vi "Plugin.Initialize.vi"(8 "error in (no error)":errorcluster, 10 "Transfers":refnum<class "DSF.Engine.Transfer.lvclass">[](array[class]), 11 "UDP Plugin in":refnum<class "UDP Plugin.lvclass">) -> (0 "error out":errorcluster, 3 "UDP Plugin out":refnum<class "UDP Plugin.lvclass">)   [LabVIEW 2017, in "UDP Plugin.lvclass"]
uses:
  UDP Plugin.lvclass
  Source/Engine/Classes/Transfer/DSF.Engine.Transfer.lvclass
  UDP Plugin.lvclass/UDP Plugin.ctl
  Source/Engine/Classes/Transfer/DSF.Engine.Transfer.lvclass/DSF.Engine.Transfer.ctl
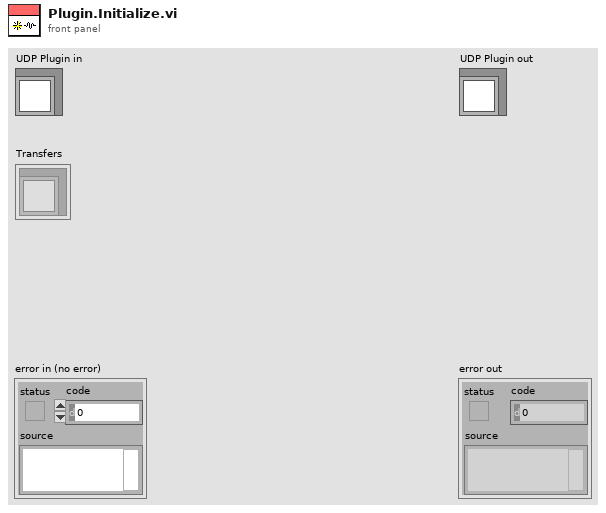
[diagram p1: front panel]
types:
  T1 = typedef "DSF.Engine.lvlib/DSF.Engine.Typedefs.ID.ctl" = i32
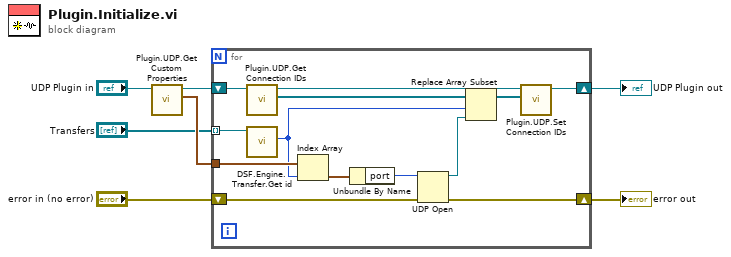
[diagram p0: block diagram]
diagram:
  n1 = call "Plugin.UDP.Get Custom Properties.vi"("UDP Plugin in"="UDP Plugin in") -> ("custom properties"=w2:cluster{"port":u16}[], "UDP Plugin out"=w3:refnum<class "UDP Plugin.lvclass">)  [unwired: 9 in]
  n2 = for {
    tunnel: "Transfers" -> [w19] mode=indexing
    tunnel: w2 -> [w18]
    shift-right: [w14] -> w6
    shift-left: w3 -> [w15]
    shift-right: [w8] -> w5
    shift-left: "error in (no error)" -> [w20]
    n3 = call "Plugin.UDP.Get Connection IDs.vi"("UDP Plugin in"=w15) -> ("connection IDs"=w12:refnum<k16>[], "UDP Plugin out"=w13:refnum<class "UDP Plugin.lvclass">)  [unwired: 9 in]
    n4 = call "DSF.Engine.Transfer.Get id.vi"("Transfer in"=w19) -> ("id"=w10:T1)  [unwired: 9 in, 1 out]
    n5 = Index Array(array=w18, index=w10) -> (element=w17:cluster{"port":u16})
    n6 = Unbundle By Name(w17) -> ("port"=w16:u16)
    n7 = UDP Open(8:w20, 11:w16) -> (port=w9:refnum<k16>, 0:w8:errorcluster)  [unwired: 3 in, 1 out]
    n8 = Replace Array Subset(array=w12, new element=w9, index=w10) -> (w11:refnum<k16>[])
    n9 = call "Plugin.UDP.Set Connection IDs.vi"("connection IDs"=w11, "UDP Plugin in"=w13) -> ("UDP Plugin out"=w14:refnum<class "UDP Plugin.lvclass">)  [unwired: 9 in]
  }
  "error out" <- w5
  "UDP Plugin out" <- w6
